vi "select-page.vi"(4 "symbol":i32, 5 "indent.lvl":i32) -> (1 "page":u16)   [LabVIEW 2015]
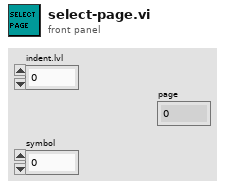
[diagram p1: front panel]
types:
  T1 = enum32{"cluster", "frame", "input.frame", "output.frame", "input.signal", "output.signal", "signal"}
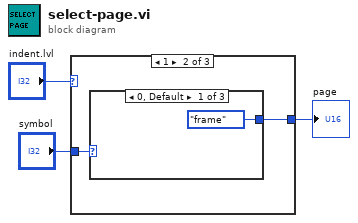
[diagram p0: block diagram]
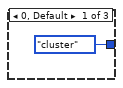
[diagram p2: hidden frame]
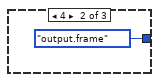
[diagram p3: hidden frame]
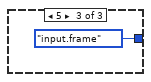
[diagram p4: hidden frame]
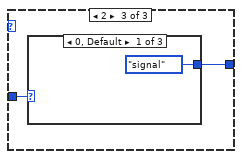
[diagram p5: hidden frame]
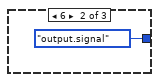
[diagram p6: hidden frame]
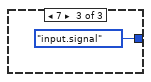
[diagram p7: hidden frame]
diagram:
  n1 = case shown="1" "indent.lvl" {
    tunnel: [T1."cluster" ("attributes") w6 w11] -> w1
    tunnel: "symbol" -> [_ w5 w10]
    frame 0, Default {
    }
    frame 1 {
      n2 = case shown="0, Default" w5 {
        tunnel: [T1."frame" ("attributes") T1."output.frame" ("attributes") T1."input.frame" ("attributes")] -> w6
        frame 0, Default {
        }
        frame 4 {
        }
        frame 5 {
        }
      }
    }
    frame 2 {
      n3 = case shown="0, Default" w10 {
        tunnel: [T1."signal" ("attributes") T1."output.signal" ("attributes") T1."input.signal" ("attributes")] -> w11
        frame 0, Default {
        }
        frame 6 {
        }
        frame 7 {
        }
      }
    }
  }
  "page" <- w1
